vi "Create Analyze Objects.vi"(7 "Reload":bool, 8 "error in (no error)":errorcluster) -> (0 "error out":errorcluster, 2 "Short Name":string[](array[string]), 3 "Objects":refnum<class "Analyze BaseClass.lvclass">[](array[class]))   [LabVIEW 2020, in "Analyze.lvlib"]
uses:
  Analyze.lvlib
  Analyze BaseClass/Analyze BaseClass.lvclass
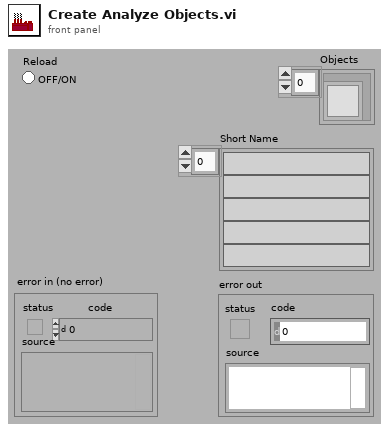
[diagram p1: front panel]
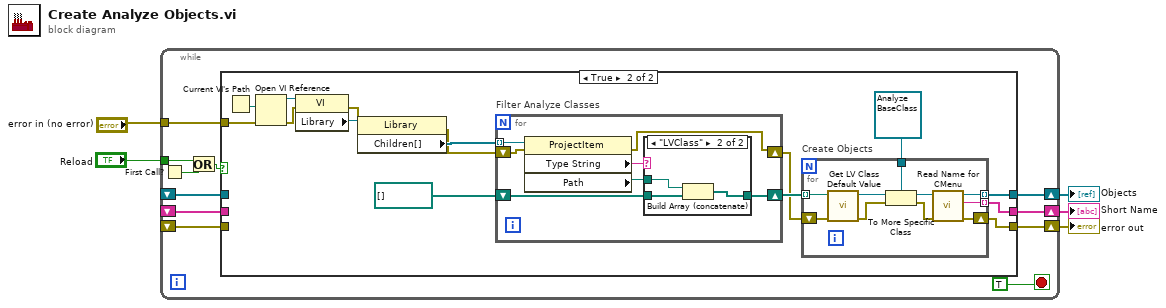
[diagram p0: block diagram]
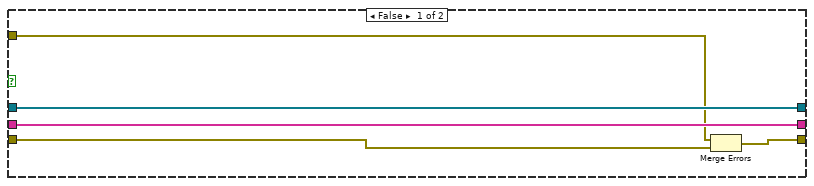
[diagram p2: hidden frame]
diagram:
  n1 = while {
    tunnel: "error in (no error)" -> [w14]
    shift-right: [w16] -> w5
    shift-left: _ -> [w8]
    shift-right: [w15] -> w4
    shift-left: _ -> [w7]
    shift-right: [w13] -> w2
    shift-left: _ -> [w6]
    tunnel: "Reload" -> [w9]
    stop <- TRUE stop-if-true
    n2 = First Call?() -> (First Call?: T/F=w11:bool)
    n3 = Or(x=w9, y=w11) -> (x .or. y?=w10:bool)
    n4 = case shown="True" w10 {
      tunnel: [w21 w31] -> w16
      tunnel: [w20 w30] -> w15
      tunnel: w14 -> [w17 w27]
      tunnel: [w18 w22] -> w13
      tunnel: w8 -> [w21 _]
      tunnel: w7 -> [w20 _]
      tunnel: w6 -> [w19 _]
      frame False {
        n5 = Merge Errors(w17, w19) -> (w18:errorcluster)
      }
      frame True {
        n6 = Current VI's Path() -> (path=w36:path)
        n7 = Open VI Reference(vi path=w36, error in (no error)=w27) -> (vi reference=w35:refnum<vi>, error out=w26:errorcluster)  [unwired: 4 in]
        n8 = property class="VI"(reference=w35, error in=w26) -> (error out=w25:errorcluster, "Library"=w34:refnum<vi>)  [unwired: 1 out]
        n9 = property class="Library"(reference=w34, error in=w25) -> (error out=w24:errorcluster, "Children[]"=w33:refnum<vi>[])  [unwired: 1 out]
        n10 = for "Filter Analyze Classes" {
          tunnel: w33 -> [w53] mode=indexing
          shift-right: [w49] -> w28
          shift-left: path[] [] -> [w51]
          shift-right: [w47] -> w23
          shift-left: w24 -> [w48]
          n11 = property class="ProjectItem"(reference=w53, error in=w48) -> (error out=w47:errorcluster, "Type String"=w52:string, "Path"=w50:path)  [unwired: 1 out]
          n12 = case shown="\"LVClass\"" w52 {
            tunnel: w51 -> [w54 w57]
            tunnel: w50 -> [_ w56]
            tunnel: [w54 w55] -> w49
            frame "False", Default {
            }
            frame "LVClass" {
              n13 = Build Array (concatenate)(w56, w57) -> (w55:path[])
            }
          }
        }
        n14 = for "Create Objects" {
          tunnel: w28 -> [w46] mode=indexing
          tunnel: [w42] -> w31 mode=indexing
          tunnel: refnum<class "Analyze BaseClass.lvclass"> refnum ("Analyze.lvlib:Analyze BaseClass.lvclass") -> [w44]
          tunnel: [w39] -> w30 mode=indexing
          shift-right: [w37] -> w22
          shift-left: w23 -> [w38]
          n15 = call <vilib>:"Get LV Class Default Value.vi"("error in (no error)"=w38, "class path"=w46) -> ("error out"=w41:errorcluster, "object"=w45:refnum<class>)  [unwired: 8 in]
          n16 = To More Specific Class(target class=w44, reference=w45, error in=w41) -> (specific class reference=w43:refnum<class "Analyze BaseClass.lvclass">, error out=w40:errorcluster)
          n17 = call-dynamic "Read Name for CMenu.vi"("error in (no error)"=w40, "Analyze BaseClass in"=w43) -> ("error out"=w37:errorcluster, "Name for Context menu"=w39:string, "Analyze BaseClass out"=w42:refnum<class "Analyze BaseClass.lvclass">)  [unwired: 7 in]
        }
      }
    }
  }
  "Objects" <- w5
  "Short Name" <- w4
  "error out" <- w2
